vi "TSM SSC Digital Write Static Per-Site Per-Pin.vi"(0 "Digital TSM In":T1, 5 "Per-Site Per-Pin State (V)":T3[][](array[typedef]) items=["0"=0, "1"=1, "X"=5], 11 "error in":errorcluster) -> (4 "Digital TSM Out":T1, 15 "error out":errorcluster)   [LabVIEW 2019]
doc: "Writes per-site per-pin static states to the specified pin(s) and pin group(s). The selected pins remain in the specified state until the next pattern burst or call to this VI. If there are uncommitted changes to levels or the termination mode, this VI commits the changes to the pins.\n\nThis VI does not change the selected pin function. If you write a static state to a pin that does not have the Digital function selected, the new static state is stored by the digital pattern instrument, and affects the state of the pin the next time you change the selected function to Digital."
uses:
  <instrlib>/niDigital/niDigital.llb/niDigital Write Static Pin State.ctl
  TSM/TSM SSC Digital.ctl
  <vilib>/NI_TestStand_SemiconductorModule/NI_TestStand_Semiconductor_Module.lvlibp/PinMap/Digital Pattern/PinQueryContext/DigitalPatternPinQueryContext.lvclass
  SSC Digital/SSC Digital.ctl
  1a9f9ff5-721a-42b6-b454-8659b893b2e8.vi
  Shared SubVIs/Trim Whitespace [Inlined].vi
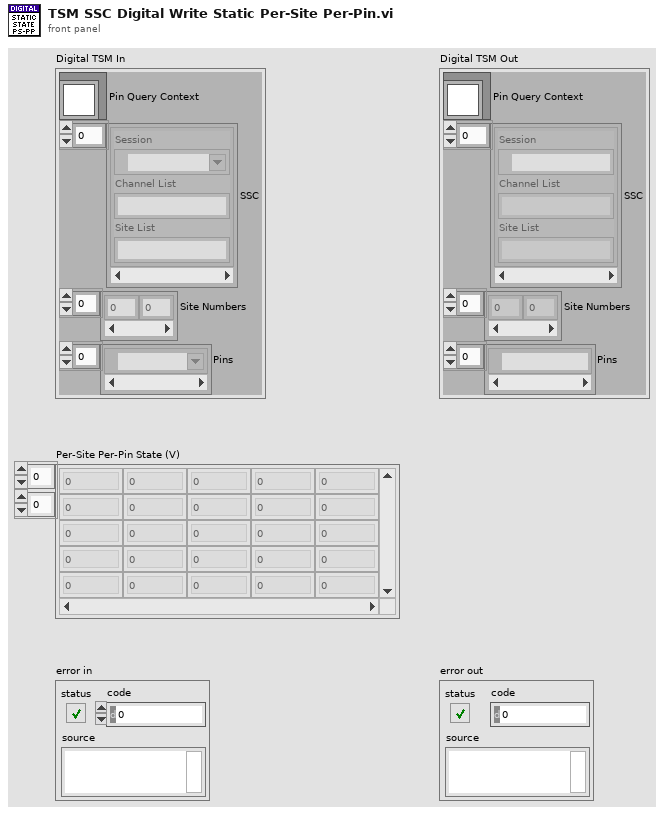
[diagram p1: front panel]
types:
  T1 = typedef "TSM SSC Digital.ctl" = cluster{"Pin Query Context":refnum<class "DigitalPatternPinQueryContext.lvclass">, "SSC":T2[], "Site Numbers":i32[], "Pins":tag[]}
  T2 = typedef "SSC Digital.ctl" = cluster{"Session":refnum<k15>, "Channel List":string, "Site List":string}
  T3 = typedef "niDigital Write Static Pin State.ctl" = u8
  T4 = typedef "Digital 2D Location.ctl" = cluster{"Row":i32, "Col":i32}
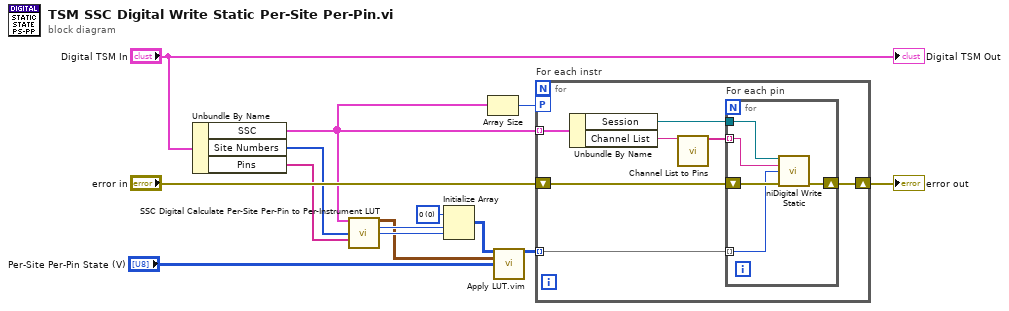
[diagram p0: block diagram]
diagram:
  w5 = T3 0 items=["0"=0, "1"=1, "X"=5] ("element")
  n1 = Unbundle By Name("Digital TSM In") -> ("SSC"=w2:T2[], "Site Numbers"=w8:i32[], "Pins"=w7:tag[])
  n2 = call "SSC Digital Calculate Per-Site Per-Pin to Per-Instrument LUT.vi"("Digital SSC In"=w2, "Sites"=w8, "Pins"=w7) -> ("Per-Site Per-Pin to Per-Instrument LUT"=w10:T4[][], "Instrument Count"=w13:i32, "Max Sites on Instrument"=w12:i32)  [unwired: 10 in]
  n3 = Initialize Array(w5, w13, w12) -> (w11:T3[][])
  n4 = Array Size(array=w2) -> (size(s)=w3:i32)
  n5 = call "Apply LUT.vim"("Initialized Array"=w11, "LUT"=w10, "Results to Apply LUT to"="Per-Site Per-Pin State (V)") -> ("Array Out"=w9:T3[][])  [unwired: 12 in]
  n6 = for "For each instr" {
    workers-P: w3 -> [_]
    tunnel: w2 -> [w16] mode=indexing
    tunnel: w9 -> [w19] mode=indexing
    shift-right: [w20] -> w4
    shift-left: "error in" -> [w21]
    n7 = Unbundle By Name(w16) -> ("Session"=w17:refnum<k15>, "Channel List"=w15:string)
    n8 = call "Channel List to Pins.vi"("Channel List"=w15) -> ("Sites and Pins"=w18:string[])  [unwired: 12 in, 2 out]
    n9 = for "For each pin" {
      shift-right: [w24] -> w20
      shift-left: w21 -> [w26]
      tunnel: w18 -> [w23] mode=indexing
      tunnel: w19 -> [w22] mode=indexing
      tunnel: w17 -> [w25]
      n10 = call <instrlib>:"niDigital Write Static.vi"("instrument handle"=w25, "channel list"=w23, "state"=w22, "error in"=w26) -> ("error out"=w24:errorcluster)  [unwired: 10 in, 1 out]
    }
  }
  "error out" <- w4
  "Digital TSM Out" <- "Digital TSM In"
